vi "Set TDMS WFM Properties.vi"(1 "Settings":string[](array[string]), 4 "Configuration":variant, 5 "dt":dbl, 6 "Scaling coefficients":dbl[][](array[numeric]), 7 "t0":dbl, 8 "error in (no error)":errorcluster, 9 "Channel names":string[](array[string]), 10 "Group name":string="p", 11 "tdms file":refnum<k34>) -> (0 "error out":errorcluster, 3 "tdms file out":refnum<k34>)   [LabVIEW 2021]
uses:
  <vilib>/Utility/tdmsutil.llb/TDMS Create Scaling Information (Linear).vi
  8a8c82c9-4748-4a37-8d6f-9f2ec094c772.vi
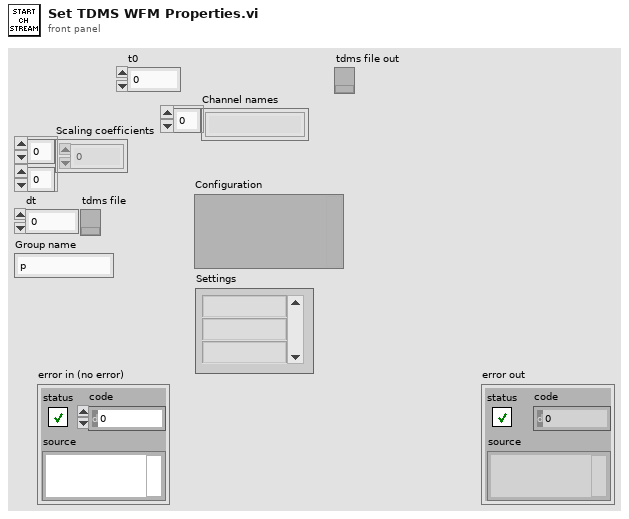
[diagram p1: front panel]
types:
  T1 = cluster{"slope":dbl, "y intercept":dbl, "input source":i32}
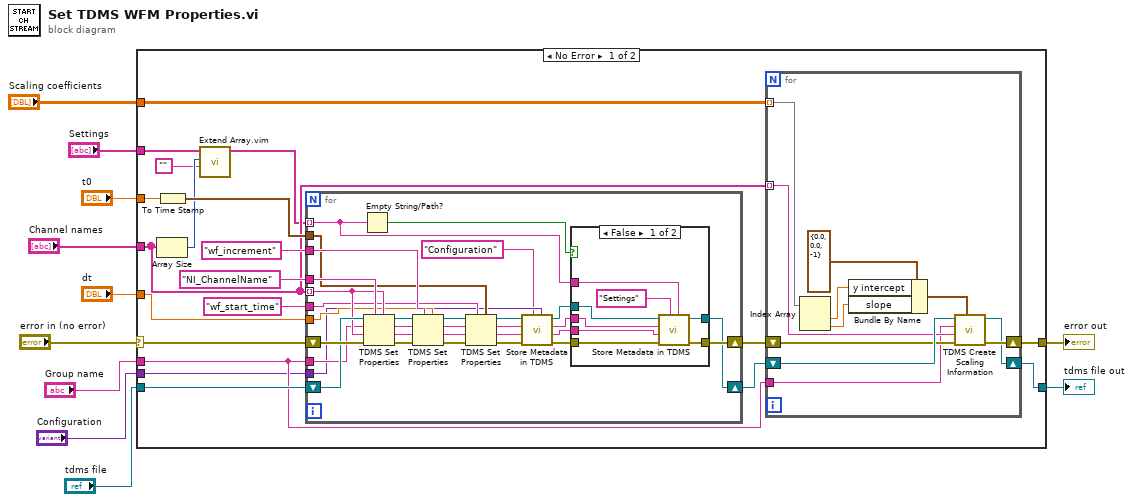
[diagram p0: block diagram]
diagram:
  n1 = case shown="No Error" "error in (no error)" {
    selector: "error in (no error)" -> [w31 w85]
    tunnel: [w19 w85] -> w10
    tunnel: "tdms file" -> [w26 w84]
    tunnel: "dt" -> [w25 _]
    tunnel: "t0" -> [w24 _]
    tunnel: "Scaling coefficients" -> [w18 _]
    tunnel: "Group name" -> [w23 _]
    tunnel: "Channel names" -> [w16 _]
    tunnel: [w20 w84] -> w3
    tunnel: "Configuration" -> [w17 _]
    tunnel: "Settings" -> [w13 _]
    frame No Error {
      n2 = Array Size(array=w16) -> (size(s)=w15:i32)
      n3 = To Time Stamp(1:w24) -> (0:w28:timestamp)
      n4 = call "Extend Array.vim"("Default value"="", "Extend to size"=w15, "Array in"=w13) -> ("Array out"=w14:string[])  [unwired: 7 in, 1 out]
      n5 = for {
        tunnel: "NI_ChannelName" -> [w70]
        tunnel: w16 -> [w69] mode=indexing
        tunnel: w25 -> [w68]
        tunnel: w28 -> [w67]
        tunnel: "wf_start_time" -> [w66]
        shift-right: [w48] -> w22
        shift-left: w31 -> [w73]
        shift-right: [w47] -> w21
        shift-left: w26 -> [w72]
        tunnel: "wf_increment" -> [w71]
        tunnel: w23 -> [w57]
        tunnel: w17 -> [w53]
        tunnel: w14 -> [w44] mode=indexing
        n6 = Empty String/Path?(string/path=w44) -> (empty?=w43:bool)
        n7 = TDMS Set Properties(5:w69, 7:w70, 8:w73, 9:w69, 10:w57, 11:w72) -> (0:w65:errorcluster, 1:w62:string, 2:w64:string, 3:w63:refnum<k34>)
        n8 = TDMS Set Properties(5:w68, 7:w71, 8:w65, 9:w62, 10:w64, 11:w63) -> (0:w61:errorcluster, 1:w60:string, 2:w59:string, 3:w58:refnum<k34>)
        n9 = TDMS Set Properties(5:w67, 7:w66, 8:w61, 9:w60, 10:w59, 11:w58) -> (0:w52:errorcluster, 1:w54:string, 2:w55:string, 3:w56:refnum<k34>)
        n10 = call "Store Metadata in TDMS.vi"("Value"=w53, "name"="Configuration" ("property names"), "Error In"=w52, "channel name"=w54, "group name"=w55, "tdms file"=w56) -> ("Error Out"=w49:errorcluster, "channel name out"=w45:string, "group name out"=w46:string, "tdms file out"=w50:refnum<k34>)  [unwired: 2 in]
        n11 = case shown="False" w43 {
          tunnel: w50 -> [w81 w83]
          tunnel: w49 -> [w80 w82]
          tunnel: [w79 w82] -> w48
          tunnel: [w78 w83] -> w47
          tunnel: w44 -> [w76 _]
          tunnel: w46 -> [w75 _]
          tunnel: w45 -> [w74 _]
          frame False {
            n12 = call "Store Metadata in TDMS.vi"("Value"=w76, "name"="Settings" ("property names"), "Error In"=w80, "channel name"=w74, "group name"=w75, "tdms file"=w81) -> ("Error Out"=w79:errorcluster, "tdms file out"=w78:refnum<k34>)  [unwired: 2 in, 2 out]
          }
          frame True {
          }
        }
      }
      n13 = for {
        tunnel: w18 -> [w40] mode=indexing
        tunnel: w16 -> [w34] mode=indexing
        shift-right: [w38] -> w19
        shift-left: w22 -> [w33]
        shift-right: [w37] -> w20
        shift-left: w21 -> [w35]
        tunnel: w23 -> [w32]
        n14 = Index Array(array=w40) -> (element #1=w42:dbl, element #2=w36:dbl)  [unwired: 2 in]
        n15 = Bundle By Name(cluster=T1 {"slope"=0.0, "y intercept"=0.0, "input source"=-1} ("linear scale"), "y intercept"=w42, "slope"=w36) -> (w41:T1)
        n16 = call-poly <vilib>:"TDMS Create Scaling Information.vi"("linear scale"=w41, "error in (no error)"=w33, "channel name"=w34, "group name"=w32, "tdms file"=w35) -> ("error out"=w38:errorcluster, "tdms file out"=w37:refnum<k34>)  [unwired: 2 in, 3 out]
      }
    }
    frame Error {
    }
  }
  "error out" <- w10
  "tdms file out" <- w3
